vi "DFD 2-Band QMF Filter Bank Design.vi"(4 "weight":dbl=0.5, 6 "fs in [Hz]":dbl=1.0, 7 "phase option":u16(ring) items=["Min-Max Phase", "Linear Phase"], 8 "error in (no error)":errorcluster, 9 "stopband attenuation [dB]":dbl=40.0, 10 "roll off":dbl=0.2, 11 "order":i32=31) -> (0 "error out":errorcluster, 2 "actual order":i32, 3 "filter bank out":T1={"mFBank_AnalysisFilters"=[], "mFBank_SynthesisFilters"=[], "mFBank_#Bands"=2, "mFBank_ProcMethod"=enum."General", "mFBank_Coeffs"=[], "mFBank_Gain"=1.0, "mFBank_Delay"=0, "mFBank_Type"=0} {"mFBank_SynthesisFilters"."mMRate_SumWl" min=1 max=32 step=1; "mFBank_SynthesisFilters"."mMRate_InputIwl" min=1 max=32 step=1; "mFBank_SynthesisFilters"."mMRate_GainWl" min=1 max=32 step=1; "mFBank_SynthesisFilters"."mMRate_OutputWl" min=1 max=32 step=1; "mFBank_SynthesisFilters"."mMRate_InputWl" min=1 max=32 step=1; "mFBank_SynthesisFilters"."mMRate_CoefWl" min=1 max=32 step=1; "mFBank_SynthesisFilters"."mMRate_Mode" items=["Default"=-1, "No Rate Change"=0, "Interpolation"=1, "Decimation"=2, "Interpolated"=3, "Rational"=4]; "mFBank_AnalysisFilters"."mMRate_SumWl" min=1 max=32 step=1; "mFBank_AnalysisFilters"."mMRate_InputIwl" min=1 max=32 step=1; "mFBank_AnalysisFilters"."mMRate_GainWl" min=1 max=32 step=1; "mFBank_AnalysisFilters"."mMRate_OutputWl" min=1 max=32 step=1; "mFBank_AnalysisFilters"."mMRate_InputWl" min=1 max=32 step=1; "mFBank_AnalysisFilters"."mMRate_CoefWl" min=1 max=32 step=1; "mFBank_AnalysisFilters"."mMRate_Mode" items=["Default"=-1, "No Rate Change"=0, "Interpolation"=1, "Decimation"=2, "Interpolated"=3, "Rational"=4]; "mFBank_Type" items=["Uniform", "Non-Uniform"]})   [LabVIEW 2017, in "NI_DigFilter_FilterBank.lvlib"]
doc: "Creates a 2-band quadrature mirror filter (QMF) filter bank."
uses:
  <vilib>/addons/Digital Filter Design/NI_DigFilter_FilterBank.lvlib
  <vilib>/addons/Digital Filter Design/FilterBank.llb/Object/DFD Filter Bank Obj.ctl
  <vilib>/addons/Digital Filter Design/_Objects.llb/DFD Multirate Filter Obj.ctl
  <vilib>/addons/Digital Filter Design/_Objects.llb/DFD Multirate Mode.ctl
  <vilib>/addons/Digital Filter Design/_Objects.llb/DFD Coef Norm Type.ctl
  <vilib>/addons/Digital Filter Design/_Objects.llb/DFD Round-off Mode.ctl
  <vilib>/addons/Digital Filter Design/_Objects.llb/DFD FXP MRate Multiply Mode.ctl
  <vilib>/addons/Digital Filter Design/FilterBank.llb/Object/DFD Filter Bank Processing Method.ctl
  <vilib>/addons/Digital Filter Design/FilterBank.llb/Object/DFD Filter Bank Type.ctl
  <vilib>/addons/Digital Filter Design/_Objects.llb/DFD Multirate Filtering Mode.ctl
  <vilib>/addons/Digital Filter Design/NI_DigFilterLicensed.lvlib
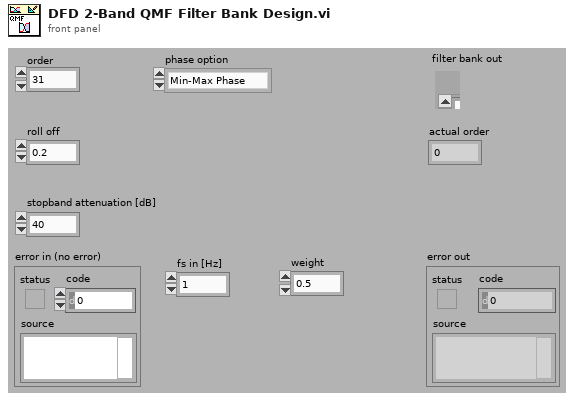
[diagram p1: front panel]
types:
  T1 = typedef "NI_DigFilter_FilterBank.lvlib/DFD Filter Bank Obj.ctl" = cluster{"mFBank_AnalysisFilters":T2[], "mFBank_SynthesisFilters":T2[], "mFBank_#Bands":i32, "mFBank_ProcMethod":T7, "mFBank_Coeffs":dbl[], "mFBank_Gain":dbl, "mFBank_Delay":i32, "mFBank_Type":T8}
  T2 = typedef "NI_DigFilterLicensed.lvlib/DFD Multirate Filter Obj.ctl" = cluster{"mMRate_Structure":enum16{"CIC", "FIR", "IIR", "Lattice"}, "mMRate_Mode":T3, "mMRate_Factor":i32, "mMRate_FIRParams":cluster{"mMRate_FIR_H":dbl[], "mMRate_FIR_IsNyquist?":bool, "mMRate_FIR_IsSymmetric?":bool}, "mMRate_CICParams":cluster{"mMRate_CIC_#Stage":i32, "mMRate_CIC_Lag":i32, "mMRate_CIC_Type":enum16{"Lowpass", "Highpass"}}, "mMRate_Order":i32, "mMRate_Version":string, "mMRate_Comments":string, "mMRate_RationalFactor":cluster{"mMRate_L":i32, "mMRate_M":i32}, "mMRate_Fs":dbl, "mMRate_Quantized?":bool, "mMRate_QFilterGain":dbl, "mMRate_CoefWl":i16, "mMRate_Scaling":cluster{"mMRate_ScaleByPowerOf2?":bool, "mMRate_ScaleType":T4}, "mMRate_InputWl":i16, "mMRate_OutputWl":i16, "mMRate_OutputMode":T5, "mMRate_MultMode":T6, "mMRate_BitPruning":bool, "mMRate_GainWl":i16, "mMRate_OutputFwl":i16, "mMRate_SumIwl":i16, "mMRate_InputIwl ":i16, "mMRate_SumWl":i16, "mMRate_CoefIwl":i16}
  T3 = typedef "NI_DigFilterLicensed.lvlib/DFD Multirate Mode.ctl" = i16
  T4 = typedef "NI_DigFilterLicensed.lvlib/DFD Coef Norm Type.ctl" = enum16{"No Norm", "Time Domain 1-Norm", "Time Domain 2-Norm", "Time Domain Inf-Norm"}
  T5 = typedef "NI_DigFilterLicensed.lvlib/DFD Round-off Mode.ctl" = enum16{"Nearest", "Truncation"}
  T6 = typedef "NI_DigFilterLicensed.lvlib/DFD FXP MRate Multiply Mode.ctl" = enum16{"Truncated", "Full"}
  T7 = typedef "NI_DigFilter_FilterBank.lvlib/DFD Filter Bank Processing Method.ctl" = enum16{"General", "2-Band QMF Lattice", "Cosine-Modulated"}
  T8 = typedef "NI_DigFilter_FilterBank.lvlib/DFD Filter Bank Type.ctl" = u16
  T9 = typedef "NI_DigFilterLicensed.lvlib/DFD Multirate Filtering Mode.ctl" = u16
  T10 = typedef "NI_DigFilter_FilterBank.lvlib/DFD Bank Obj.ctl" = cluster{"mBank_Filters":T2[], " mBank_#Bands":i32, "mBank_ProcMethod":T7, "mBank_Coeffs":dbl[], "mBank_Gain":dbl, "mBank_Type":T8}
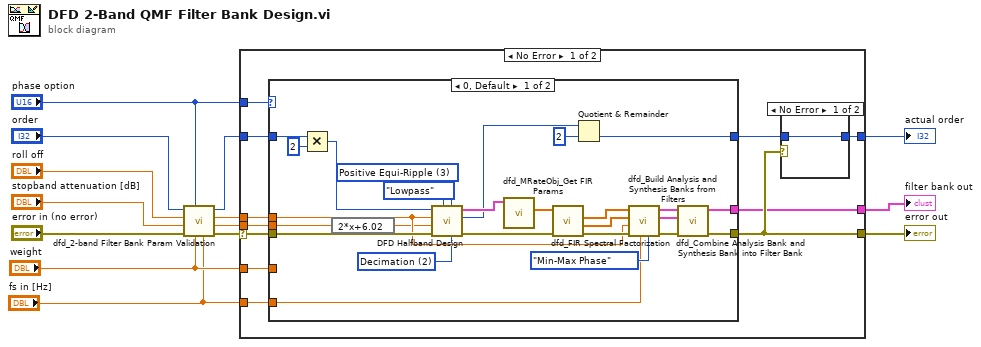
[diagram p0: block diagram]
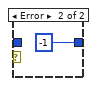
[diagram p2: hidden frame]
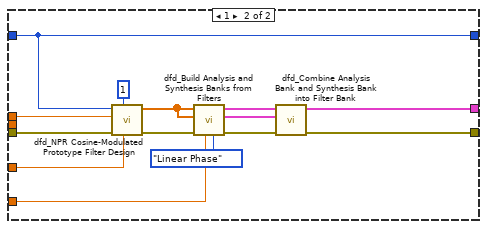
[diagram p3: hidden frame]
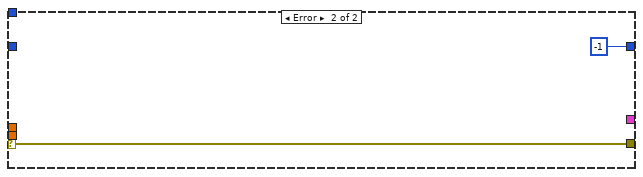
[diagram p4: hidden frame]
diagram:
  n1 = call <vilib>:"dfd_2-band Filter Bank Param Validation.vi"("fs in [Hz]"="fs in [Hz]", "weight"="weight", "phase option"="phase option", "error in (no error)"="error in (no error)", "stopband attenuation [dB]"="stopband attenuation [dB]", "roll off"="roll off", "order"="order") -> ("error out"=w2:errorcluster, "dup stopband attenuation [dB]"=w3:dbl, "dup roll off"=w5:dbl, "dup order"=w4:i32)  [unwired: 1 in]
  n2 = case shown="No Error" w2 {
    selector: w2 -> [w16 w69]
    tunnel: "phase option" -> [w25 _]
    tunnel: [w24 w69] -> w11
    tunnel: [w23 -1 ("order")] -> w10
    tunnel: [w22 _] -> w8
    tunnel: "weight" -> [w21 _]
    tunnel: w5 -> [w19 _]
    tunnel: w4 -> [w18 _]
    tunnel: w3 -> [w17 _]
    tunnel: "fs in [Hz]" -> [w15 _]
    frame No Error {
      n3 = case shown="0, Default" w25 {
        tunnel: w16 -> [w49 w67]
        tunnel: w19 -> [w32 w65]
        tunnel: w17 -> [w29 _]
        tunnel: [w35 w59] -> w24
        tunnel: [w34 w61] -> w22
        tunnel: [w36 w64] -> w20
        tunnel: w18 -> [w43 w64]
        tunnel: w21 -> [_ w55]
        tunnel: w15 -> [w28 w54]
        frame 0, Default {
          w31 = T9 2 items=["No Rate Change", "Interpolation", "Decimation"] ("filtering mode")
          w46 = u16 3 items=["Kaiser Window", "Dolph-Chebyshev Window", "Equi-Ripple", "Positive Equi-Ripple", "Max Flat"] ("method")
          n4 = Multiply(x=w43, y=2) -> (x*y=w42:i32)
          n5 = expression code="2*x+6.02"(w29) -> (w30:dbl)
          n6 = call <vilib>:"DFD Halfband Design.vi"("filtering mode"=w31, "method"=w46, "filter type"=enum16{"Lowpass", "Highpass"}."Lowpass", "error in (no error)"=w49, "stopband attenuation [dB]"=w30, "roll off"=w32, "order"=w42) -> ("error out"=w50:errorcluster, "order out"=w33:i32, "multirate filter out"=w44:T2)  [unwired: 2 in]
          n7 = call <vilib>:"dfd_MRateObj_Get FIR Params.vi"("multirate filter in"=w44) -> ("h(n)"=w39:dbl[])  [unwired: 7 in, 3 out]
          n8 = call <vilib>:"dfd_FIR Spectral Factorization.vi"("error in (no error)"=w50, "H(n)"=w39) -> ("error out"=w37:errorcluster, "H(n) 2"=w47:dbl[], "H(n) 1"=w38:dbl[])  [unwired: 7 in]
          n9 = Quotient & Remainder(x=w33, y=2) -> (floor(x/y)=w36:i32)  [unwired: 1 out]
          n10 = call <vilib>:"dfd_Build Analysis and Synthesis Banks from Filters.vi"("phase option"=enum16{"Min-Max Phase", "Linear Phase"}."Min-Max Phase", "fs"=w28, "error in (no error)"=w37, "roll-off"=w32, "F 0"=w47, "H 0"=w38) -> ("error out"=w53:errorcluster, "synthesis bank"=w51:T10, "analysis bank"=w52:T10)  [unwired: 3 in]
          n11 = call <vilib>:"dfd_Combine Analysis Bank and Synthesis Bank into Filter Bank.vi"("error in (no error)"=w53, "synthesis bank"=w51, "analysis bank"=w52) -> ("error out"=w35:errorcluster, "filter bank out"=w34:T1)  [unwired: 7 in]
        }
        frame 1 {
          n12 = call <vilib>:"dfd_NPR Cosine-Modulated Prototype Filter Design.vi"("weight"=w55, "band counts"=1 ("number of bands"), "error in (no error)"=w67, "roll off"=w65, "order"=w64) -> ("error out"=w58:errorcluster, "h"=w56:dbl[])  [unwired: 5 in]
          n13 = call <vilib>:"dfd_Build Analysis and Synthesis Banks from Filters.vi"("phase option"=enum16{"Min-Max Phase", "Linear Phase"}."Linear Phase", "fs"=w54, "error in (no error)"=w58, "F 0"=w56, "H 0"=w56) -> ("error out"=w60:errorcluster, "synthesis bank"=w62:T10, "analysis bank"=w63:T10)  [unwired: 4 in]
          n14 = call <vilib>:"dfd_Combine Analysis Bank and Synthesis Bank into Filter Bank.vi"("error in (no error)"=w60, "synthesis bank"=w62, "analysis bank"=w63) -> ("error out"=w59:errorcluster, "filter bank out"=w61:T1)  [unwired: 7 in]
        }
      }
      n15 = case shown="No Error" w24 {
        tunnel: w20 -> [w26 _]
        tunnel: [w26 -1 ("order")] -> w23
        frame No Error {
        }
        frame Error {
        }
      }
    }
    frame Error {
    }
  }
  "error out" <- w11
  "filter bank out" <- w8
  "actual order" <- w10
